vi "New649DigitGen.vi"(2 "const + StdAvr":dbl) -> (0 "2D ResUArr - STD of each row is equal to (Last STD - Avr STD)":u64[][](array[numeric]), 1 "Waveform Graph":dbl[][](graph), 3 "CurrAvrSTDToArr - only six":dbl[](array[numeric]))   [LabVIEW 2023]
panel:
  out "size(s)":i32
  out "Size(s)":i32
  out "Last STD":dbl format="%#_3g"
  out "Avr STD":dbl
  out "Std":dbl[](array[numeric]) format="%#_4g"
  out "AvrSTDtoArray - All":dbl[](array[numeric]) format="%#_4g"
  out "LastSTDToArray":dbl[](array[numeric])
  out "Row Std":dbl[](array[numeric]) format="%#_3f"
  out "Java file - official result":i64[][](array[numeric])
  # "Генерира масив всеки ред на който е с STD = AvrResultsSTD +/- N"
  # "K"
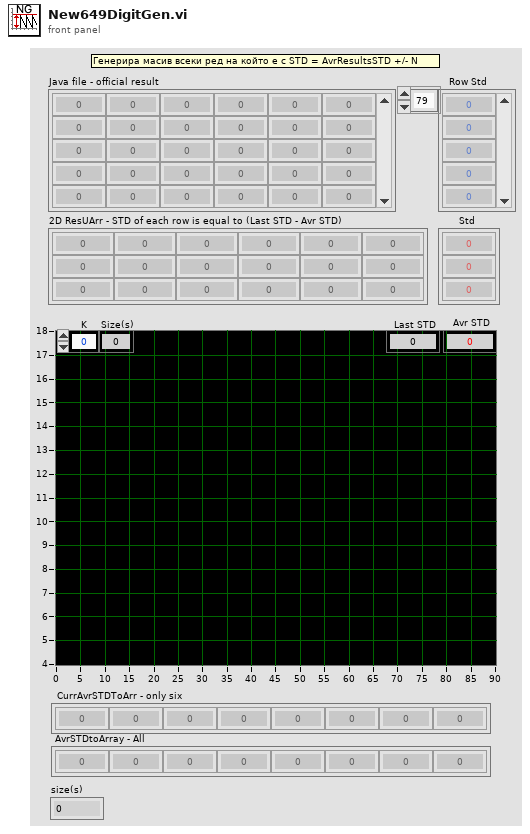
[diagram p1: front panel]
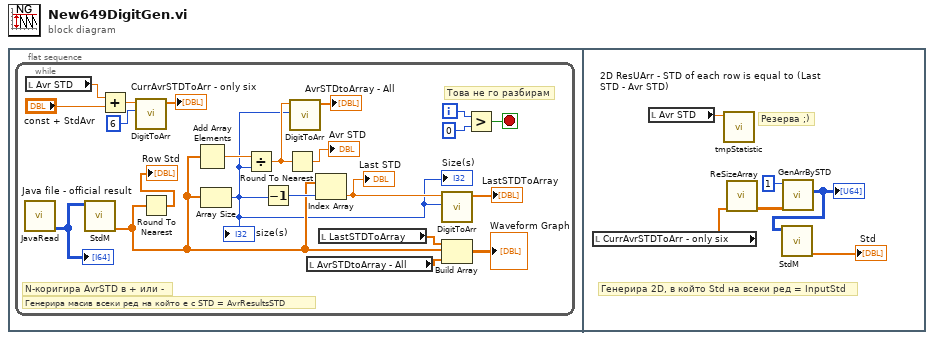
[diagram p0: block diagram]
diagram:
  n1 = flat-sequence {
    frame #0 {
      n2 = while {
        i -> [w11]
        stop <- w9 stop-if-true
        # "Това не го разбирам"
        # "N-коригира AvrSTD в + или -"
        # "Генерира масив всеки ред на който е с STD = AvrResultsSTD"
        n3 = call "JavaRead.vi"() -> ("Java file"=w22:i64[][])  [unwired: 10 in, 1 out]
        "Java file - official result" <- w22
        n4 = local read "Avr STD"() -> (w4:dbl)
        n5 = call "StdM.vi"("2D in"=w22) -> ("1D Std"=w6:dbl[])  [unwired: 6 in, 4 out]
        n6 = Add(x=w4, y="const + StdAvr") -> (x+y=w1:dbl)
        n7 = call "DigitToArr.vi"("Arr Size"=6, "Digit"=w1) -> ("Array out"=→"CurrAvrSTDToArr - only six":dbl[])  [unwired: 9 in]
        n8 = Round To Nearest(number=w6) -> (nearest integer value=→"Row Std":dbl[])
        n9 = Add Array Elements(numeric array=w6) -> (sum=w21:dbl)
        n10 = Array Size(array=w6) -> (size(s)=w2:i32)
        "Size(s)" <- w2
        "size(s)" <- w2
        n11 = Divide(x=w21, y=w2) -> (x/y=w8:dbl)
        n12 = Decrement(x=w2) -> (x-1=w19:i32)
        n13 = Round To Nearest(number=w8) -> (nearest integer value=→"Avr STD":dbl)
        n14 = call "DigitToArr.vi"("Arr Size"=w2, "Digit"=w8) -> ("Array out"=→"AvrSTDtoArray - All":dbl[])  [unwired: 9 in]
        n15 = local read "AvrSTDtoArray - All"() -> (w14:dbl[])
        n16 = Index Array(array=w6, index=w19) -> (element=w18:dbl)
        "Last STD" <- w18
        n17 = local read "LastSTDToArray"() -> (w15:dbl[])
        n18 = call "DigitToArr.vi"("Arr Size"=w2, "Digit"=w18) -> ("Array out"=→"LastSTDToArray":dbl[])  [unwired: 9 in]
        n19 = Build Array(w15, w6, w14) -> (→"Waveform Graph":dbl[][])
        n20 = Greater?(x=w11, y=0) -> (0:w9:bool)
      }
    }
    frame #1 {
      # "Генерира 2D, в който Std на всеки ред = InputStd"
      # "Резерва ;)"
      n21 = local read "CurrAvrSTDToArr - only six"() -> (w24:dbl[])
      n22 = local read "Avr STD"() -> (w28:dbl)
      n23 = call "tmpStatistic.vi"("My Std"=w28) -> ()  [unwired: 10 in, 1 out]
      n24 = call "ReSizeArray.vi"("1D"=w24) -> ("2D"=w27:dbl[][])  [unwired: 9 in, 1 out]
      n25 = call "GenArrBySTD.vi"("2D Array"=w27, "Last idx -"=1) -> ("2D ResUArr"=w25:u64[][])  [unwired: 6 in, 3 out]
      "2D ResUArr - STD of each row is equal to (Last STD - Avr STD)" <- w25
      n26 = call "StdM.vi"("2D in"=w25) -> ("1D Std"=→"Std":dbl[])  [unwired: 6 in, 4 out]
    }
  }
